vi "Linkages NodeID to GUID.vi"(7 "Command/Response Refnum in":T1 format="%.0x", 8 "error in (no error)":errorcluster, 11 "Linked Channels in":T2[](array[typedef]) {"Channel Refnum" format="%.0x"}) -> (0 "error out":errorcluster, 3 "Linked Channels out":cluster{"Variable Name":string, "GUID":string}[](array[cluster]))   [LabVIEW 2018, in "Instrument Addon Scripting API.lvlib"]
uses:
  Instrument Addon Scripting API.lvlib
  TypeDefs/Linked Channel.ctl
  <vilib>/NI Veristand/Custom Device API/Custom Device Item Ref.ctl
  <vilib>/NI/NI VeriStand Advanced SysDef API/_SubVIs/SysDef.Search.Parent.vi
  Addon/Addon Shared/SubVIs/Constants.vi
  Addon/Addon Shared/Instrument Addon Shared.lvlib
  <vilib>/NI/NI VeriStand Advanced SysDef API/SysDef API/Advanced System Definition.lvlib
  <vilib>/NI Veristand/Custom Device API/Custom Device API.lvlib
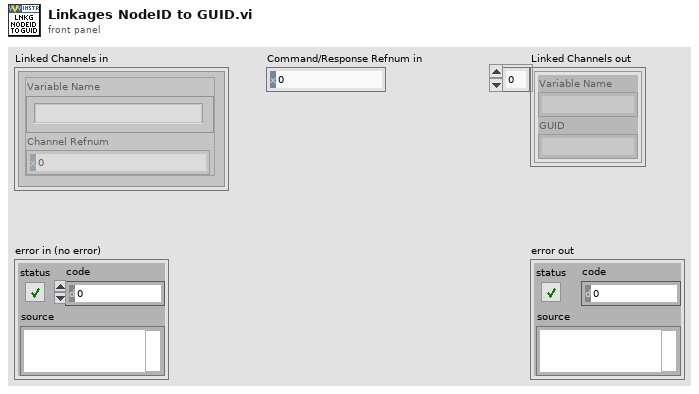
[diagram p1: front panel]
types:
  T1 = typedef "Custom Device API.lvlib/Custom Device Item Ref.ctl" = u64
  T2 = typedef "Instrument Addon Scripting API.lvlib/Linked Channel.ctl" = cluster{"Variable Name":string, "Channel Refnum":T1}
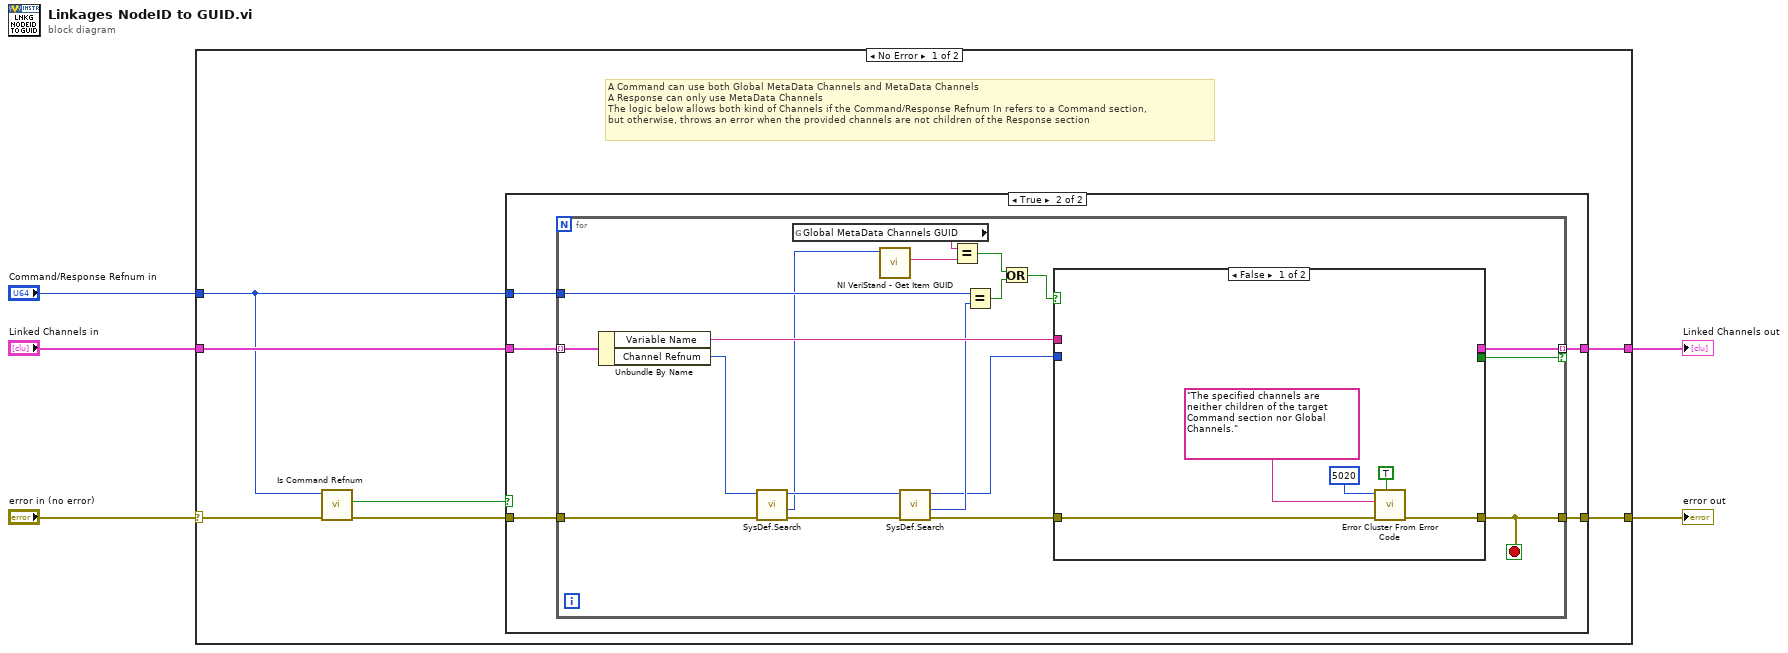
[diagram p0: block diagram]
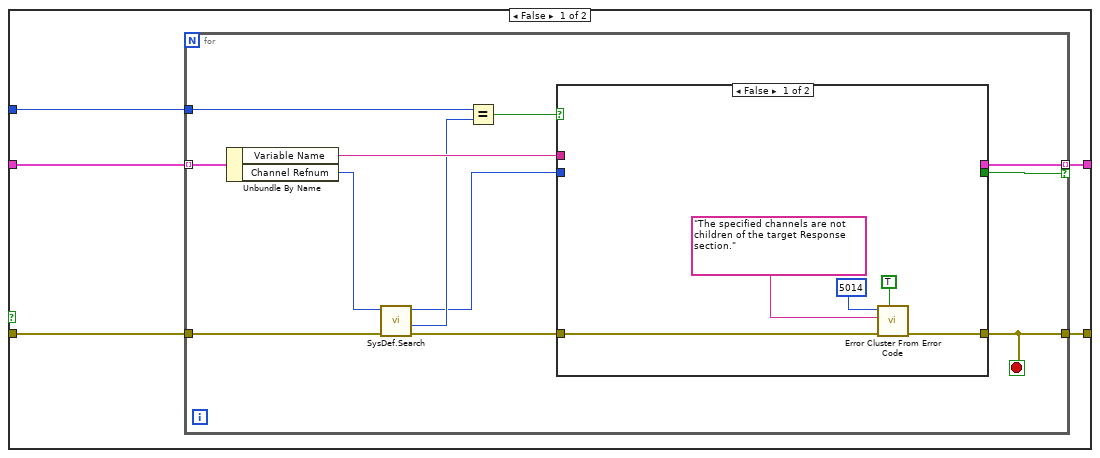
[diagram p2: hidden frame]
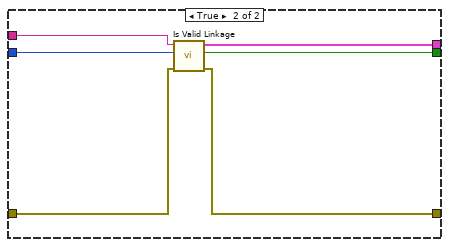
[diagram p3: hidden frame]
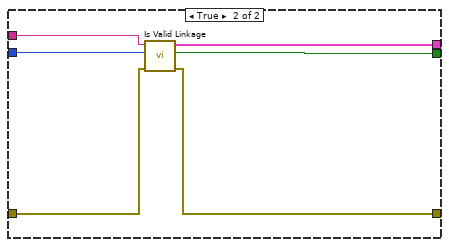
[diagram p4: hidden frame]
diagram:
  n1 = case shown="No Error" "error in (no error)" {
    selector: "error in (no error)" -> [w7 w76]
    tunnel: [w12 _] -> w5
    tunnel: [w11 w76] -> w4
    tunnel: "Linked Channels in" -> [w10 _]
    tunnel: "Command/Response Refnum in" -> [w9 _]
    frame No Error {
      # "A Command can use both Global MetaData Channels and MetaData Channels\nA Response can only use MetaData Channels\nThe logic below allows both kind of Channels if the Command/Response Refnum In refers to a Command section, \nbut otherwise, throws an error when the provided channels are not children of the Response section"
      n2 = call "Is Command Refnum.vi"("error in (no error)"=w7, "Command/Response Refnum in"=w9) -> ("error out"=w6:errorcluster, "Is Command?"=w8:bool)  [unwired: 7 in, 1 out]
      n3 = case shown="True" w8 {
        tunnel: [w17 w42] -> w12
        tunnel: [w16 w41] -> w11
        tunnel: w10 -> [w15 w44]
        tunnel: w6 -> [w14 w43]
        tunnel: w9 -> [w13 w45]
        frame False {
          n4 = for {
            tunnel: w15 -> [w29] mode=indexing
            tunnel: w14 -> [w18]
            tunnel: [w27] -> w17 mode=indexing if=w26
            tunnel: [w25] -> w16
            tunnel: w13 -> [w20]
            stop <- w25 stop-if-true
            n5 = Unbundle By Name(w29) -> ("Variable Name"=w28:string, "Channel Refnum"=w24:T1)
            n6 = call-poly <vilib>:"SysDef.Search.vi"("error in (no error)"=w18, "nodeID"=w24) -> ("error out"=w22:errorcluster, "Value out"=w23:u64, "nodeID out"=w21:u64)  [unwired: 6 in, 1 out]
            n7 = Equal?(x=w20, y=w23) -> (x = y?=w19:bool)
            n8 = case shown="False" w19 {
              tunnel: w28 -> [_ w39]
              tunnel: [_ w38] -> w27
              tunnel: [_ w37] -> w26
              tunnel: [w33 w35] -> w25
              tunnel: w22 -> [w34 w36]
              tunnel: w21 -> [_ w40]
              frame False {
                n9 = call <vilib>:"Error Cluster From Error Code.vi"("show call chain? (False)"=TRUE, "error in (no error)"=w34, "error message (\"\")"="The specified channels are not children of the target Response section." ("error message (\"\")"), "error code (0)"=5014) -> ("error out"=w33:errorcluster)  [unwired: 5 in]
              }
              frame True {
                n10 = call "Is Valid Linkage.vi"("error in (no error)"=w36, "Channel Refnum"=w40, "Variable Name"=w39) -> ("error out"=w35:errorcluster, "Is Valid Linkage?"=w37:bool, "Linkage"=w38:cluster{"Variable Name":string, "GUID":string})  [unwired: 6 in]
              }
            }
          }
        }
        frame True {
          n11 = for {
            tunnel: w44 -> [w64] mode=indexing
            tunnel: w43 -> [w49]
            tunnel: [w62] -> w42 mode=indexing if=w61
            tunnel: [w60] -> w41
            tunnel: w45 -> [w56]
            stop <- w60 stop-if-true
            n12 = Unbundle By Name(w64) -> ("Variable Name"=w63:string, "Channel Refnum"=w50:T1)
            n13 = call-poly <vilib>:"SysDef.Search.vi"("error in (no error)"=w49, "nodeID"=w50) -> ("error out"=w47:errorcluster, "Value out"=w46:u64, "nodeID out"=w48:u64)  [unwired: 6 in, 1 out]
            n14 = global read "Constants.vi" "Global MetaData Channels GUID"() -> (w54:string)
            n15 = call <vilib>:"NI VeriStand - Get Item GUID.vi"("Item Ref in"=w46) -> ("GUID"=w55:string)  [unwired: 8 in, 2 out]
            n16 = call-poly <vilib>:"SysDef.Search.vi"("error in (no error)"=w47, "nodeID"=w48) -> ("error out"=w58:errorcluster, "Value out"=w59:u64, "nodeID out"=w57:u64)  [unwired: 6 in, 1 out]
            n17 = Equal?(x=w54, y=w55) -> (x = y?=w52:bool)
            n18 = Equal?(x=w56, y=w59) -> (x = y?=w53:bool)
            n19 = Or(x=w52, y=w53) -> (x .or. y?=w51:bool)
            n20 = case shown="False" w51 {
              tunnel: w63 -> [_ w75]
              tunnel: [_ w70] -> w62
              tunnel: [_ w71] -> w61
              tunnel: [w68 w72] -> w60
              tunnel: w58 -> [w69 w73]
              tunnel: w57 -> [_ w74]
              frame False {
                n21 = call <vilib>:"Error Cluster From Error Code.vi"("show call chain? (False)"=TRUE, "error in (no error)"=w69, "error message (\"\")"="The specified channels are neither children of the target Command section nor Global Channels." ("error message (\"\")"), "error code (0)"=5020) -> ("error out"=w68:errorcluster)  [unwired: 5 in]
              }
              frame True {
                n22 = call "Is Valid Linkage.vi"("error in (no error)"=w73, "Channel Refnum"=w74, "Variable Name"=w75) -> ("error out"=w72:errorcluster, "Is Valid Linkage?"=w71:bool, "Linkage"=w70:cluster{"Variable Name":string, "GUID":string})  [unwired: 6 in]
              }
            }
          }
        }
      }
    }
    frame Error {
    }
  }
  "Linked Channels out" <- w5
  "error out" <- w4
